vi "Get measurementservice_DMMConfigResponse.vi"(8 "error in (no error)":errorcluster, 11 "gRPCid":T3) -> (0 "error out":errorcluster, 2 "Message Data":T1, 3 "gRPCid out":T3)   [LabVIEW 2019, in "HVC2.lvlib" / "HVC2.lvclass"]
uses:
  HVC2.lvclass
  gRPC lvSupport/Server API/typeDefs/grpcId.ctl
  measurementservice_DMMConfigResponse_Data.ctl
  measurementservice_ErrorOut/measurementservice_ErrorOut_Data.ctl
  a51dd2a7-b5c1-4c09-9df4-8cd9d3bd0c19.vi
  gRPC lvSupport/Server API/Server/Get Server DLL Path.vi
  gRPC lvSupport/gprc-lvsupport.lvlib
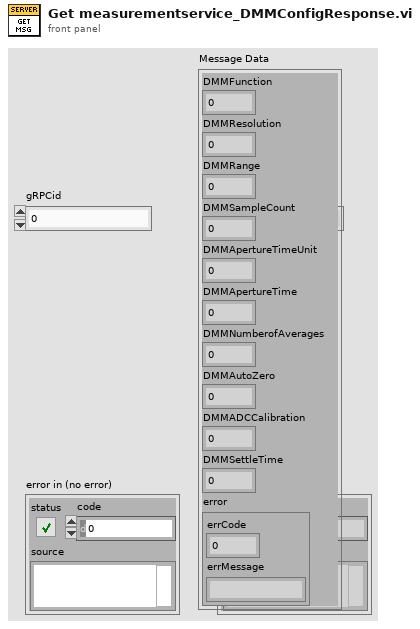
[diagram p1: front panel]
types:
  T1 = typedef "HVC2.lvlib/HVC2.lvclass/measurementservice_DMMConfigResponse_Data.ctl" = cluster{"DMMFunction":i32, "DMMResolution":sgl, "DMMRange":sgl, "DMMSampleCount":i32, "DMMApertureTimeUnit":i32, "DMMApertureTime":sgl, "DMMNumberofAverages":i32, "DMMAutoZero":i32, "DMMADCCalibration":i32, "DMMSettleTime":sgl, "error":T2}
  T2 = typedef "HVC2.lvlib/HVC2.lvclass/measurementservice_ErrorOut_Data.ctl" = cluster{"errCode":i32, "errMessage":string}
  T3 = typedef "HVC2.lvlib/gprc-lvsupport.lvlib/grpcId.ctl" = u64
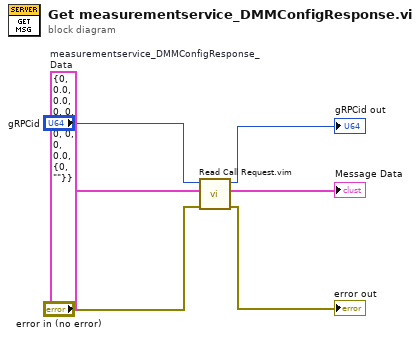
[diagram p0: block diagram]
diagram:
  w2 = T1 {"DMMFunction"=0, "DMMResolution"=0.0, "DMMRange"=0.0, "DMMSampleCount"=0, "DMMApertureTimeUnit"=0, "DMMApertureTime"=0.0, "DMMNumberofAverages"=0, "DMMAutoZero"=0, "DMMADCCalibration"=0, "DMMSettleTime"=0.0, "error"={"errCode"=0, "errMessage"=""}}  # measurementservice_DMMConfigResponse_Data
  n1 = call "Read Call Request.vim"("error in (no error)"="error in (no error)", "Data Type"=w2, "gRPCid in"="gRPCid") -> ("error out"=→"error out":errorcluster, "Request Data"=→"Message Data":T1, "gRPCid out"=→"gRPCid out":T3)  [unwired: 6 in]
